vi "Read local bitfile path.vi"(8 "error in":errorcluster, 11 "Targets in":refnum<class "Targets.lvclass">) -> (0 "error out":errorcluster, 2 "bitfile path":path, 3 "Targets out":refnum<class "Targets.lvclass">)   [LabVIEW 2013, in "PL Framework Configuration Tool.lvlib" / "Targets.lvclass"]
uses:
  Targets.lvclass
  Targets.lvclass/Targets.ctl
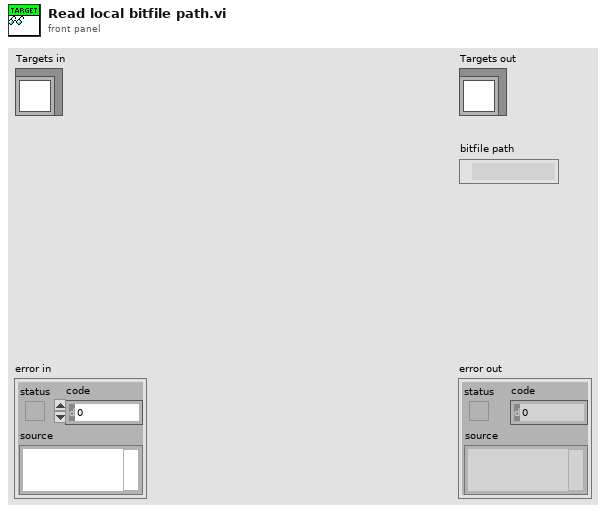
[diagram p1: front panel]
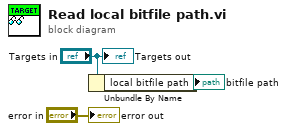
[diagram p0: block diagram]
diagram:
  n1 = Unbundle By Name("Targets in") -> ("local bitfile path"=→"bitfile path":path)
  "error out" <- "error in"
  "Targets out" <- "Targets in"
